vi "Read Text File Sink Configuration.vi"(11 "Text File Sink in":refnum<class "Text File Sink.lvclass">) -> (2 "Text File Sink Configuration":T1, 3 "Text File Sink out":refnum<class "Text File Sink.lvclass">)   [LabVIEW 2016, in "Stream Log.lvlib" / "Text File Sink.lvclass"]
uses:
  <userlib>/Composed Systems/Stream/Log/Text File Sink/Text File Sink.lvclass
  <userlib>/Composed Systems/Stream/Log/Text File Sink/Configuration.ctl
  <userlib>/Composed Systems/Stream/Log/Text File Sink/Text File Sink.lvclass/Text File Sink.ctl
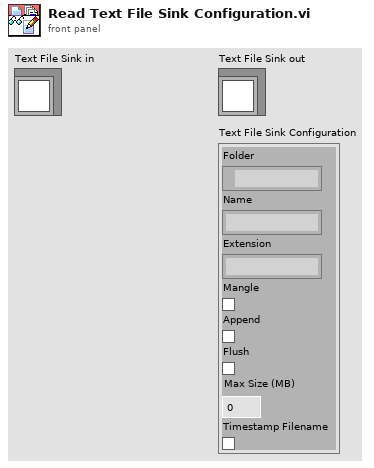
[diagram p1: front panel]
types:
  T1 = typedef "Stream Log.lvlib/Text File Sink.lvclass/Configuration.ctl" = cluster{"Folder":path, "Name":string, "Extension":string, "Mangle":bool, "Append":bool, "Flush":bool, "Max Size (MB)":i64, "Timestamp Filename":bool}
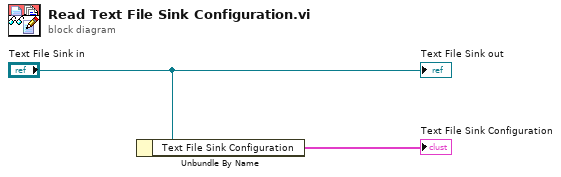
[diagram p0: block diagram]
diagram:
  n1 = Unbundle By Name("Text File Sink in") -> ("Text File Sink Configuration"=→"Text File Sink Configuration":T1)
  "Text File Sink out" <- "Text File Sink in"
